vi "DCPowerInstrument_CallCreateSessionsWithUnregisteredSessionsReserved_RemoteSessionsCreated.vi"(8 "error in":errorcluster) -> (0 "error out":errorcluster, 2 "result":string, 3 "pass":bool)   [LabVIEW 2020, in "MeasurementServerTests.lvlib"]
uses:
  MeasurementServerTests.lvlib
  78c0f8c1-8fe2-4936-9d85-28ac64cefb56.vi
  Runtime/MeasurementLink niDCPower/Create Sessions - NSess.vi
  Runtime/MeasurementLink Session Management/Session Reservation/Session Reservation.lvclass
  Runtime/MeasurementLink niDCPower/MeasurementLink niDCPower.lvlib
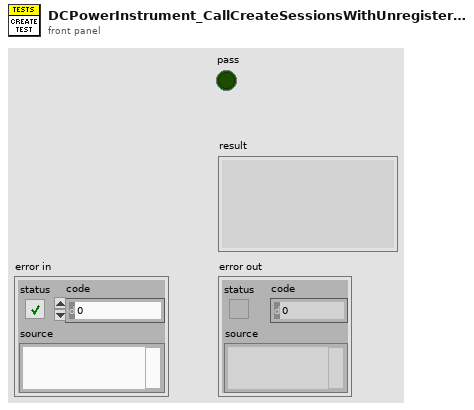
[diagram p1: front panel]
types:
  T1 = typedef "MeasurementLink Session Management.lvlib/Session Reservation.lvclass/Data.ctl" = cluster{"session and driver infos":T2[]}
  T2 = typedef "MeasurementLink Session Management.lvlib/Session Reservation.lvclass/Session and Driver Info.ctl" = cluster{"session info":T3, "session":variant}
  T3 = typedef "MeasurementLink Session Management Client.lvlib/ni_measurementlink_sessionmanagement_v1_SessionInformation.ctl" = cluster{"session":T4, "resource_name":string, "channel_list":string, "instrument_type_id":string, "session_exists":bool, "channel_mappings":T5[]}
  T4 = typedef "MeasurementLink Session Management Client.lvlib/nidevice_grpc_Session.ctl" = cluster{"name":string}
  T5 = typedef "MeasurementLink Session Management Client.lvlib/ni_measurementlink_sessionmanagement_v1_ChannelMapping.ctl" = cluster{"pin_or_relay_name":string, "site":i32, "channel":string}
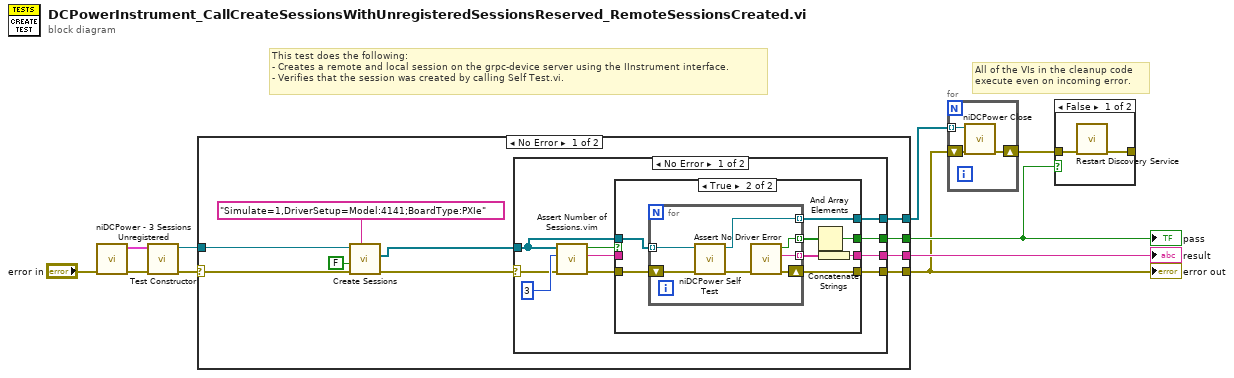
[diagram p0: block diagram]
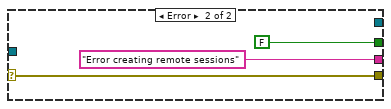
[diagram p3: hidden frame]
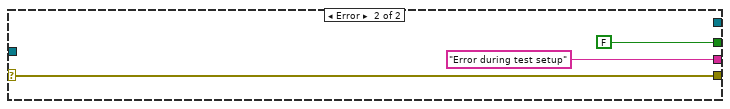
[diagram p4: hidden frame]
diagram:
  # "All of the VIs in the cleanup code\nexecute even on incoming error."
  # "This test does the following:\n- Creates a remote and local session on the grpc-device server using the IInstrument interface.\n- Verifies that the session was created by calling Self Test.vi."
  n1 = call "niDCPower - 3 Sessions Unregistered.vi"("error in"="error in") -> ("error out"=w4:errorcluster, "data out"=w5:T1)  [unwired: 9 in]
  n2 = call "Test Constructor.vi"("error in"=w4, "data"=w5) -> ("error out"=w2:errorcluster, "Session Reservation out"=w1:refnum<class "Session Reservation.lvclass">)  [unwired: 8 in]
  n3 = case shown="No Error" w2 {
    selector: w2 -> [w15 w53]
    tunnel: [w19 w53] -> w6
    tunnel: [w20 FALSE] -> w7
    tunnel: [w18 "Error during test setup" ("f")] -> w10
    tunnel: [w17 _] -> w9
    tunnel: w1 -> [w16 _]
    frame No Error {
      n4 = call-poly "Create Sessions.vi"("option string"="Simulate=1,DriverSetup=Model:4141;BoardType:PXIe", "error in"=w15, "reset"=FALSE, "session reservation in"=w16) -> ("error out"=w12:errorcluster, "sessions"=w11:refnum<k15>[])  [unwired: 4 in, 2 out]
      n5 = case shown="No Error" w12 {
        selector: w12 -> [w24 w51]
        tunnel: [w25 FALSE] -> w20
        tunnel: [w29 w51] -> w19
        tunnel: [w30 "Error creating remote sessions"] -> w18
        tunnel: [w28 _] -> w17
        tunnel: w11 -> [w27 _]
        frame No Error {
          n6 = call "Assert Number of Sessions.vim"("error in"=w24, "expected number of sessions"=3 ("y"), "sessions"=w27) -> ("error out"=w23:errorcluster, "result"=w21:string, "pass"=w22:bool)  [unwired: 6 in]
          n7 = case shown="True" w22 {
            selector: w22 -> [w34 _]
            tunnel: [w33 w35] -> w30
            tunnel: [w32 w40] -> w29
            tunnel: [w31 w39] -> w28
            tunnel: w27 -> [w31 w38]
            tunnel: [w34 w36] -> w25
            tunnel: w23 -> [w32 w37]
            tunnel: w21 -> [w33 _]
            frame False {
            }
            frame True {
              n8 = for {
                tunnel: [w49] -> w42 mode=indexing
                tunnel: [w48] -> w41 mode=indexing
                tunnel: [w46] -> w39 mode=indexing
                tunnel: w38 -> [w44] mode=indexing
                shift-right: [w47] -> w40
                shift-left: w37 -> [w43]
                n9 = call <instrlib>:"niDCPower Self Test.vi"("error in (no error)"=w43, "instrument handle"=w44) -> ("error out"=w45:errorcluster, "instrument handle out"=w46:refnum<k15>)  [unwired: 6 in, 2 out]
                n10 = call "Assert No Driver Error.vi"("error in"=w45) -> ("error out"=w47:errorcluster, "result"=w48:string, "pass?"=w49:bool)  [unwired: 8 in]
              }
              n11 = And Array Elements(Boolean array=w42) -> (logical AND=w36:bool)
              n12 = Concatenate Strings(w41) -> (w35:string)
            }
          }
        }
        frame Error {
        }
      }
    }
    frame Error {
    }
  }
  "error out" <- w6
  "pass" <- w7
  "result" <- w10
  n13 = for {
    tunnel: w9 -> [w58] mode=indexing
    shift-right: [w57] -> w8
    shift-left: w6 -> [w56]
    n14 = call <instrlib>:"niDCPower Close.vi"("error in (no error)"=w56, "instrument handle"=w58) -> ("error out"=w57:errorcluster)  [unwired: 9 in]
  }
  n15 = case shown="False" w7 {
    tunnel: w8 -> [w60 _]
    tunnel: [w59 _] -> _
    frame False {
      n16 = call "Restart Discovery Service.vi"("error in"=w60) -> ("error out"=w59:errorcluster)  [unwired: 10 in]
    }
    frame True {
    }
  }
